vi "Get_MPUTemp.vi"(5 "Device Number":T1, 7 "Update":bool) -> (2 "MPUTemp":dbl)   [LabVIEW 2016]
doc: "This navX VI returns the current MPU Temperature."
uses:
  <vilib>/Rock Robotics/WPI/NavX/_TypeDefs/FRIC_navX_DeviceNumbersTypeDef.ctl
  <vilib>/Rock Robotics/WPI/NavX/_TypeDefs/Z900_navX_DeviceRegisters.ctl
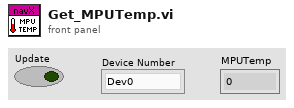
[diagram p1: front panel]
types:
  T1 = typedef "FRIC_navX_DeviceNumbersTypeDef.ctl" = enum16{"Dev0", "Dev1", "Dev2", "Dev3", "Dev4", "Dev5", "Dev6", "Dev7", "Dev8", "Dev9", "Dev10"}
  T2 = typedef "Z900_navX_DeviceRegisters.ctl" = u8
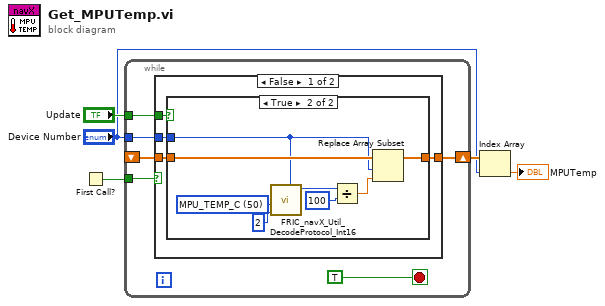
[diagram p0: block diagram]
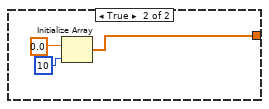
[diagram p3: hidden frame]
diagram:
  n1 = First Call?() -> (First Call?: T/F=w4:bool)
  n2 = while {
    shift-right: [w11] -> w3
    shift-left: _ -> [w8]
    tunnel: "Update" -> [w9]
    tunnel: "Device Number" -> [w7]
    tunnel: w4 -> [w6]
    stop <- TRUE stop-if-true
    n3 = case shown="False" w6 {
      tunnel: [w15 w27] -> w11
      tunnel: w9 -> [w14 _]
      tunnel: w8 -> [w13 _]
      tunnel: w7 -> [w12 _]
      frame False {
        n4 = case shown="True" w14 {
          tunnel: [w16 w19] -> w15
          tunnel: w13 -> [w16 w20]
          tunnel: w12 -> [_ w17]
          frame False {
          }
          frame True {
            w22 = T2 50 items=["WHOAMI"=0, "HW_REV"=1, "FW_VER_MAJOR"=2, "FW_VER_MINOR"=3, "UPDATE_RATE_HZ"=4, "ACCEL_FSR_G"=5, "GYRO_FSR_DPS"=6, "OP_STATUS"=8, "CAL_STATUS"=9, "SELFTEST_STATUS"=10, "CAPABILITY_FLAGS_L"=11, "CAPABILITY_FLAGS_H"=12, "SENSOR_STATUS"=16, "TIMESTAMP"=18, "YAW"=22, "ROLL"=24, "PITCH"=26, "HEADING"=28, "FUSED_HEADING"=30, "ALTITUDE_I"=32, "ALTITUDE_D"=34, "LINERA_ACC_X"=36, "LINERA_ACC_Y"=38, "LINERA_ACC_Z"=40, "QUAT_W"=42, "QUAT_X"=44, "QUAT_Y"=46, "QUAT_Z"=48, "MPU_TEMP_C"=50, "GYRO_X"=52, "GYRO_Y"=54, "GYRO_Z"=56, "ACC_X"=58, "ACC_Y"=60, "ACC_Z"=62, "MAG_X"=64, "MAG_Y"=66, "MAG_Z"=68, "PRESSURE_I"=70, "PRESSURE_D"=72, "PRESSURE_TEMP"=74, "YAW_OFFSET"=76, "QUAT_OFFSET_W"=78, "QUAT_OFFSET_X"=80, "QUAT_OFFSET_Y"=82, "QUAT_OFFSET_Z"=84, "INTEGRATION_CONTROL"=86, "VELOCITY_X"=88, "VELOCITY_Y"=92, "VELOCITY_Z"=96, "DISPLACMENT_X"=100, "DISPLACMENT_Y"=104, "DISPLACEMENT_Z"=108] ("Device Register")
            n5 = call <vilib>:"FRIC_navX_Util_DecodeProtocol_Int16.vi"("Device Number"=w17, "length"=2, "Device Register"=w22) -> ("Value"=w23:i16)  [unwired: 8 in]
            n6 = Divide(x=w23, y=100) -> (x/y=w18:dbl)
            n7 = Replace Array Subset(array=w20, new element=w18, index=w17) -> (w19:dbl[])
          }
        }
      }
      frame True {
        n8 = Initialize Array(0.0, 10 ("dimension size")) -> (w27:dbl[])
      }
    }
  }
  n9 = Index Array(array=w3, index="Device Number") -> (element=→"MPUTemp":dbl)
